vi "Check Path.vi"(10 "Library Path":path, 11 "lvzstd in":refnum<class "lvzstd.lvclass">) -> (0 "error in (no error)":errorcluster, 3 "output lvzstd":refnum<class "lvzstd.lvclass">)   [LabVIEW 2020, in "lvzstd.lvlib" / "lvzstd.lvclass"]
uses:
  lvzstd.lvclass
  lvzstd.lvclass/lvzstd.ctl
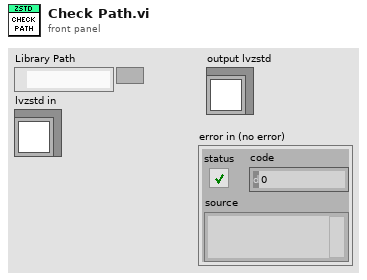
[diagram p1: front panel]
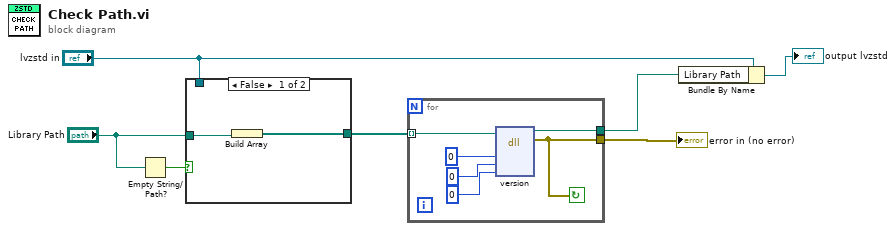
[diagram p0: block diagram]
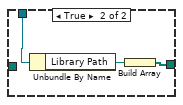
[diagram p2: hidden frame]
diagram:
  n1 = Empty String/Path?(string/path="Library Path") -> (empty?=w6:bool)
  n2 = case shown="False" w6 {
    tunnel: "lvzstd in" -> [_ w12]
    tunnel: [w8 w10] -> w4
    tunnel: "Library Path" -> [w9 _]
    frame False {
      n3 = Build Array(w9) -> (w8:path[])
    }
    frame True {
      n4 = Unbundle By Name(w12) -> ("Library Path"=w11:path)
      n5 = Build Array(w11) -> (w10:path[])
    }
  }
  n6 = for {
    tunnel: w4 -> [w15] mode=indexing
    tunnel: [w14] -> w3
    tunnel: [w13] -> w2
    stop <- w14 continue-if-true
    n7 = dll-call lib="?" fn="version"(path in=w15, "major"=0, "minor"=0, "patch"=0) -> (path out=w13:path, error out=w14:errorcluster)  [unwired: 6 in]
  }
  "error in (no error)" <- w3
  n8 = Bundle By Name(cluster="lvzstd in", "Library Path"=w2) -> (→"output lvzstd":refnum<class "lvzstd.lvclass">)
